vi "Make 1 wire.vi"(8 "error in":errorcluster, 10 "Wire Terminal 2":refnum<vi>, 11 "Wire Terminal 1":refnum<vi>) -> (0 "error out":errorcluster, 2 "Wire":refnum<vi>, 3 "Wire Sink Terminal Out":refnum<vi>)   [LabVIEW 2014, in "Scripting Tools.lvlib"]
doc: "Connects a wire between the two terminals, working out which is source and which is sink. If one or other terminal is not a valid reference, then does not make a wire. Returns a reference to the sink terminal if a wire was successfully made."
uses:
  <userlib>/_LAVACR/Scripting Tools/Scripting Tools.lvlib
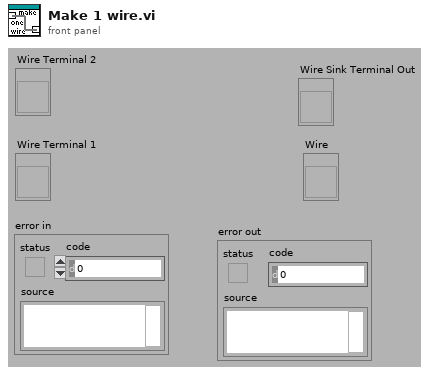
[diagram p1: front panel]
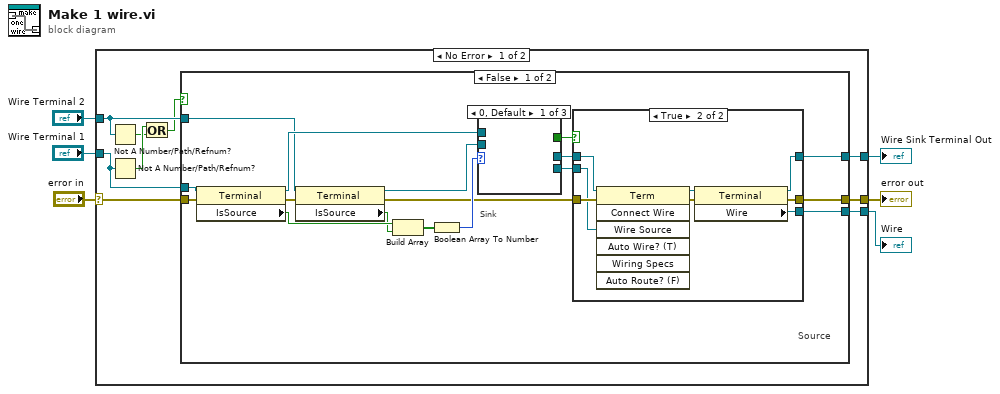
[diagram p0: block diagram]
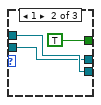
[diagram p2: hidden frame]
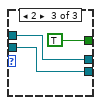
[diagram p3: hidden frame]
diagram:
  n1 = case shown="No Error" "error in" {
    selector: "error in" -> [w13 w50]
    tunnel: [w15 w50] -> w6
    tunnel: "Wire Terminal 2" -> [w9 _]
    tunnel: [w14 _] -> w4
    tunnel: "Wire Terminal 1" -> [w10 _]
    tunnel: [w7 _] -> w1
    frame No Error {
      n2 = Not A Number/Path/Refnum?(number/path/refnum=w9) -> (NaN/Path/Refnum?=w11:bool)
      n3 = Not A Number/Path/Refnum?(number/path/refnum=w10) -> (NaN/Path/Refnum?=w12:bool)
      n4 = Or(x=w12, y=w11) -> (x .or. y?=w8:bool)
      n5 = case shown="False" w8 {
        tunnel: [w32 w49] -> w15
        tunnel: [w31 _] -> w14
        tunnel: w13 -> [w30 w49]
        tunnel: w10 -> [w22 _]
        tunnel: w9 -> [w21 _]
        tunnel: [w16 _] -> w7
        frame False {
          # "Sink"
          # "Source"
          n6 = property class="Terminal"(reference=w22, error in=w30) -> (reference out=w24:refnum<vi>, error out=w29:errorcluster, "IsSource"=w28:bool)
          n7 = property class="Terminal"(reference=w21, error in=w29) -> (reference out=w23:refnum<vi>, error out=w20:errorcluster, "IsSource"=w27:bool)
          n8 = Build Array(w28, w27) -> (w26:bool[])
          n9 = Boolean Array To Number(Boolean array=w26) -> (number=w25:u32)
          n10 = case shown="0, Default" w25 {
            tunnel: w24 -> [_ w35 w37]
            tunnel: w23 -> [_ w34 w38]
            tunnel: [_ w35 w38] -> w19
            tunnel: [_ w34 w37] -> w18
            tunnel: [_ TRUE TRUE] -> w17
            frame 0, Default {
            }
            frame 1 {
            }
            frame 2 {
            }
          }
          n11 = case shown="True" w17 {
            tunnel: [w40 w43] -> w32
            tunnel: w20 -> [w40 w48]
            tunnel: w18 -> [w39 w47]
            tunnel: w19 -> [_ w46]
            tunnel: [w39 w42] -> w31
            tunnel: [_ w41] -> w16
            frame False {
            }
            frame True {
              n12 = invoke class="Term" method="Connect Wire"(reference=w47, error in=w48, "Wire Source"=w46) -> (reference out=w45:refnum<vi>, error out=w44:errorcluster)  [unwired: 4 in, 5 out]
              n13 = property class="Terminal"(reference=w45, error in=w44) -> (reference out=w42:refnum<vi>, error out=w43:errorcluster, "Wire"=w41:refnum<vi>)
            }
          }
        }
        frame True {
        }
      }
    }
    frame Error {
    }
  }
  "error out" <- w6
  "Wire Sink Terminal Out" <- w4
  "Wire" <- w1
